vi "solar_type Get Value (Binary).vi"(8 "error in (no error)":errorcluster, 9 "Position (0,-1=LVDefault)":cluster{"Bit_Offset":i32, "Bit_Size":i32}={"Bit_Offset"=0, "Bit_Size"=-1}, 10 "Variant":variant, 11 "Buffered Data (Binary)":string) -> (0 "error out":errorcluster, 1 "New Offset":i32, 2 "Value (Binary)":string, 3 "Buffered Data out (Binary)":string, 5 "LVType":T1)   [LabVIEW 2018]
doc: "This gets the flattened binary value from the variant and inserts it into the 'Buffered Data' string.\nNote: The buffered data string must be padded with the appropriate string size."
uses:
  solar_type Item Type.ctl
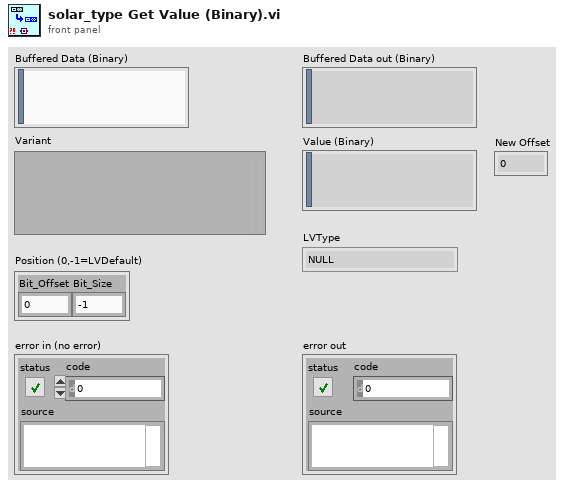
[diagram p1: front panel]
types:
  T1 = typedef "solar_type Item Type.ctl" = enum16{"NULL", "UNKNOWN", "CLUSTER", "I8", "I16", "I32", "I64", "U8", "U16", "U32", "U64", "U8_ENUM", "U16_ENUM", "U32_ENUM", "SGL", "DBL", "BOOLEAN", "STRING", "PATH", "VISA", "TAG", "TIME", "I8_1D", "I16_1D", "I32_1D", "I64_1D", "U8_1D", "U16_1D", "U32_1D", "U64_1D", "U8_ENUM_1D", "U16_ENUM_1D", "U32_ENUM_1D", "SGL_1D", "DBL_1D", "BOOLEAN_1D", "STRING_1D", "PATH_1D", "VISA_1D", "TAG_1D", "TIME_1D", "I8_2D", "I16_2D", "I32_2D", "I64_2D", "U8_2D", "U16_2D", "U32_2D", "U64_2D", "U8_ENUM_2D", "U16_ENUM_2D", "U32_ENUM_2D", "SGL_2D", "DBL_2D", "BOOLEAN_2D", "STRING_2D", "PATH_2D", "VISA_2D", "TAG_2D", "TIME_2D"}
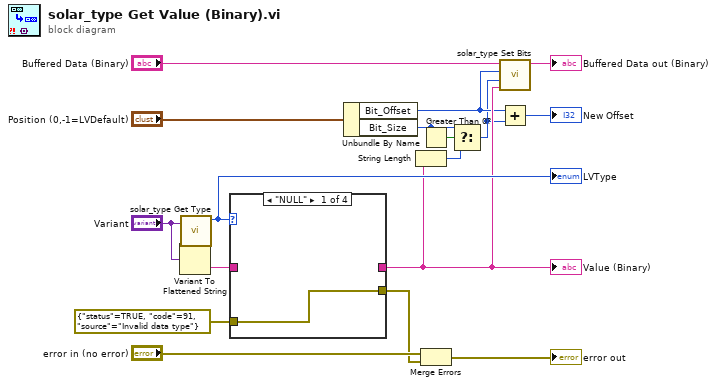
[diagram p0: block diagram]
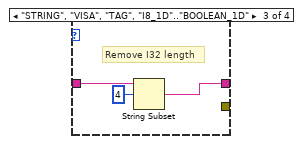
[diagram p3: hidden frame]
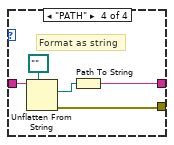
[diagram p4: hidden frame]
diagram:
  n1 = Variant To Flattened String(Variant="Variant") -> (data string=w13:string)  [unwired: 1 out]
  n2 = call "solar_type Get Type.vi"("Variant"="Variant") -> ("Type"=w14:T1)  [unwired: 4 in, 2 out]
  "LVType" <- w14
  n3 = case shown="\"NULL\"" w14 {
    tunnel: w13 -> [_ w19 w22 w27]
    tunnel: [_ w19 w20 w23] -> w6
    tunnel: [w18 _ _ w25] -> w12
    tunnel: errorcluster {"status"=TRUE, "code"=91, "source"="Invalid data type"} ("error in (no error)") -> [w18 _ _ _]
    frame "NULL" {
    }
    frame Default {
      # "BLOCK"
    }
    frame "STRING", "VISA", "TAG", "I8_1D".."BOOLEAN_1D" {
      # "Remove I32 length"
      n4 = String Subset(string=w22, offset (0)=4) -> (substring=w20:string)  [unwired: 1 in]
    }
    frame "PATH" {
      # "Format as string"
      n5 = Unflatten From String(type=path "", binary string=w27) -> (value=w24:path, error out=w25:errorcluster)  [unwired: 3 in, 1 out]
      n6 = Path To String(path=w24) -> (string=w23:string)
    }
  }
  "Value (Binary)" <- w6
  n7 = Unbundle By Name("Position (0,-1=LVDefault)") -> ("Bit_Offset"=w3:i32, "Bit_Size"=w4:i32)
  n8 = String Length(string=w6) -> (length=w5:i32)
  n9 = Greater Than 0?(x=w4) -> (x > 0?=w7:bool)
  n10 = Merge Errors("error in (no error)", w12) -> (→"error out":errorcluster)
  n11 = Select(t=w4, s=w7, f=w5) -> (s? t:f=w2:i32)
  n12 = call "solar_type Set Bits.vi"("Value (Binary)"=w6, "Bit Size (32)"=w2, "Bit Offset (0)"=w3, "Buffered Data in"="Buffered Data (Binary)") -> ("Buffered Data with Value"=→"Buffered Data out (Binary)":string)  [unwired: 7 in]
  n13 = Add(x=w3, y=w2) -> (x+y=→"New Offset":i32)
